vi "release_resources.vi"(8 "error in (no error)":errorcluster, 11 "LabJackRes":T1) -> (0 "error out":errorcluster)   [LabVIEW 2025, in "LabJackEKG.lvlib"]
uses:
  LabJackEKG.lvlib
  Typedefs/LabJackGlobalResources.ctl
  Typedefs/CounterQueues.ctl
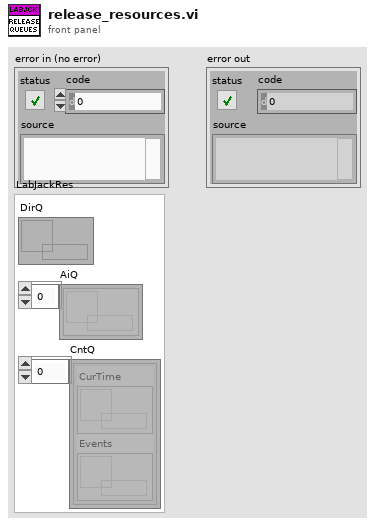
[diagram p1: front panel]
types:
  T1 = typedef "LabJackEKG.lvlib/LabJackGlobalResources.ctl" = cluster{"DirQ":refnum<queue>, "AiQ":refnum<queue>[], "CntQ":T2[]}
  T2 = typedef "LabJackEKG.lvlib/CounterQueues.ctl" = cluster{"CurTime":refnum<queue>, "Events":refnum<queue>}
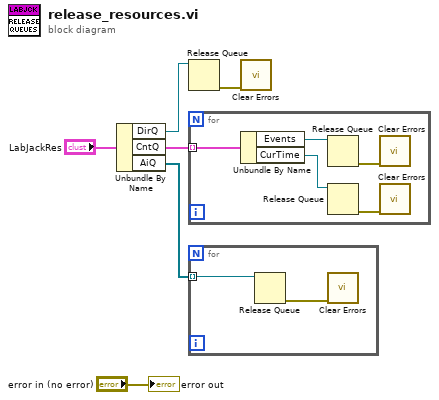
[diagram p0: block diagram]
diagram:
  n1 = Unbundle By Name("LabJackRes") -> ("DirQ"=w5:refnum<queue>, "CntQ"=w4:T2[], "AiQ"=w3:refnum<queue>[])
  n2 = Release Queue(queue=w5) -> (error out=w2:errorcluster)  [unwired: 2 in, 2 out]
  n3 = for {
    tunnel: w4 -> [w10] mode=indexing
    n4 = Unbundle By Name(w10) -> ("Events"=w9:refnum<queue>, "CurTime"=w8:refnum<queue>)
    n5 = Release Queue(queue=w9) -> (error out=w11:errorcluster)  [unwired: 2 in, 2 out]
    n6 = Release Queue(queue=w8) -> (error out=w7:errorcluster)  [unwired: 2 in, 2 out]
    n7 = call <vilib>:"Clear Errors.vi"("error in (no error)"=w11) -> ()  [unwired: 5 in, 2 out]
    n8 = call <vilib>:"Clear Errors.vi"("error in (no error)"=w7) -> ()  [unwired: 5 in, 2 out]
  }
  n9 = for {
    tunnel: w3 -> [w12] mode=indexing
    n10 = Release Queue(queue=w12) -> (error out=w13:errorcluster)  [unwired: 2 in, 2 out]
    n11 = call <vilib>:"Clear Errors.vi"("error in (no error)"=w13) -> ()  [unwired: 5 in, 2 out]
  }
  n12 = call <vilib>:"Clear Errors.vi"("error in (no error)"=w2) -> ()  [unwired: 5 in, 2 out]
  "error out" <- "error in (no error)"
